vi "GetSonarPower (SubVI).vi"() -> (3 "Value":dbl format="%#_13g")   [LabVIEW 2017]
uses:
  <vilib>/Rock Robotics/WPI/Solenoid/WPI_SolenoidValue.ctl
  <vilib>/Rock Robotics/WPI/Ultrasonic/WPI_SonarMB1010AnalogRefNum Registry Get.vi
  <vilib>/Rock Robotics/WPI/Solenoid/WPI_SolenoidSetEnum.vi
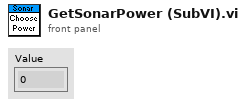
[diagram p1: front panel]
types:
  T1 = typedef "WPI_SonarMB1010AnalogDeviceRef.ctl" = cluster{"AIDeviceRef":T2, "Scaling factor (V/in)":dbl, "Average Bits":u8}
  T2 = typedef "WPI_AnalogChannelDevRef.ctl" = cluster{"DevStatus":errorcluster, "Analog Channel":T3}
  T3 = typedef "FPGA_AIChannel.ctl" = enum8{"AI 0", "AI 1", "AI 2", "AI 3", "AI MXP 0", "AI MXP 1", "AI MXP 2", "AI MXP 3", "Invalid"}
  T4 = typedef "WPI_SolenoidValue.ctl" = enum16{"Off", "On", "Forward", "Reverse"}
  T5 = typedef "WPI_SolenoidDevRef.ctl" = cluster{"DevStatus":errorcluster, "Pneumatics Control Module":u8, "Forward Solenoid Channel":T6, "Reverse Solenoid Channel":T6}
  T6 = typedef "WPI_SolenoidChannel.ctl" = enum8{"Solenoid 0", "Solenoid 1", "Solenoid 2", "Solenoid 3", "Solenoid 4", "Solenoid 5", "Solenoid 6", "Solenoid 7", "Invalid"}
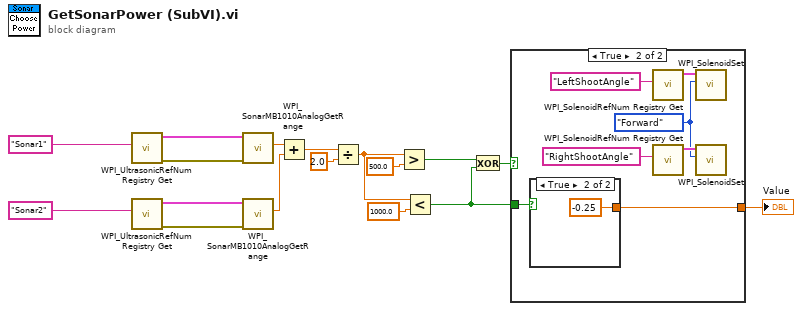
[diagram p0: block diagram]
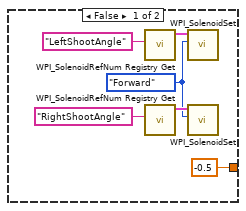
[diagram p2: hidden frame]
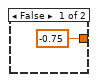
[diagram p3: hidden frame]
diagram:
  n1 = call-poly <vilib>:"WPI_UltrasonicRefNum Registry Get.vi"("refnum name"="Sonar1") -> ("error out"=w4:errorcluster, "SonarMB1010AnalogDevRef"=w5:T1)  [unwired: 9 in]
  n2 = call-poly <vilib>:"WPI_UltrasonicRefNum Registry Get.vi"("refnum name"="Sonar2") -> ("error out"=w7:errorcluster, "SonarMB1010AnalogDevRef"=w8:T1)  [unwired: 9 in]
  n3 = call "WPI_SonarMB1010AnalogGetRange.vi"("error in"=w4, "SonarMB1010AnalogDevRef"=w5) -> ("Distance"=w3:dbl)  [unwired: 7 in, 2 out]
  n4 = call "WPI_SonarMB1010AnalogGetRange.vi"("error in"=w7, "SonarMB1010AnalogDevRef"=w8) -> ("Distance"=w6:dbl)  [unwired: 7 in, 2 out]
  n5 = Add(x=w3, y=w6) -> (x+y=w17:dbl)
  n6 = Divide(x=w17, y=2.0) -> (x/y=w14:dbl)
  n7 = Greater?(x=w14, y=500.0) -> (0:w11:bool)
  n8 = Less?(x=w14, y=1000.0) -> (x < y?=w10:bool)
  n9 = Exclusive Or(1:w10, 2:w11) -> (0:w12:bool)
  n10 = case shown="True" w12 {
    tunnel: w10 -> [_ w30]
    tunnel: [-0.5 w29] -> w9
    frame False {
      w20 = WPI_SolenoidValue."Forward" ("Value")
      n11 = call <vilib>:"WPI_SolenoidRefNum Registry Get.vi"("refnum name"="LeftShootAngle") -> ("SolenoidDevRef"=w18:T5)  [unwired: 9 in, 1 out]
      n12 = call <vilib>:"WPI_SolenoidRefNum Registry Get.vi"("refnum name"="RightShootAngle") -> ("SolenoidDevRef"=w22:T5)  [unwired: 9 in, 1 out]
      n13 = call-poly <vilib>:"WPI_SolenoidSet.vi"("Value"=w20, "SolenoidDevRef"=w18) -> ()  [unwired: 8 in, 2 out]
      n14 = call-poly <vilib>:"WPI_SolenoidSet.vi"("Value"=w20, "SolenoidDevRef"=w22) -> ()  [unwired: 8 in, 2 out]
    }
    frame True {
      w25 = WPI_SolenoidValue."Forward" ("Value")
      n15 = case shown="True" w30 {
        tunnel: [-0.75 -0.25] -> w29
        frame False {
        }
        frame True {
        }
      }
      n16 = call <vilib>:"WPI_SolenoidRefNum Registry Get.vi"("refnum name"="LeftShootAngle") -> ("SolenoidDevRef"=w24:T5)  [unwired: 9 in, 1 out]
      n17 = call <vilib>:"WPI_SolenoidRefNum Registry Get.vi"("refnum name"="RightShootAngle") -> ("SolenoidDevRef"=w27:T5)  [unwired: 9 in, 1 out]
      n18 = call-poly <vilib>:"WPI_SolenoidSet.vi"("Value"=w25, "SolenoidDevRef"=w24) -> ()  [unwired: 8 in, 2 out]
      n19 = call-poly <vilib>:"WPI_SolenoidSet.vi"("Value"=w25, "SolenoidDevRef"=w27) -> ()  [unwired: 8 in, 2 out]
    }
  }
  "Value" <- w9
